vi "DB Execute.vi"(7 "table Name":string, 8 "error in (no error)":errorcluster, 11 "Db Reference":refnum<k24>) -> (0 "error out":errorcluster, 2 "Data":string[][](array[string]), 3 "Db Reference":refnum<k24>)   [LabVIEW 2020]
uses:
  D:/Labview/Auto Run Screen/Source Code/Database/Support/dbquery.dll
  Support/dbquery.dll
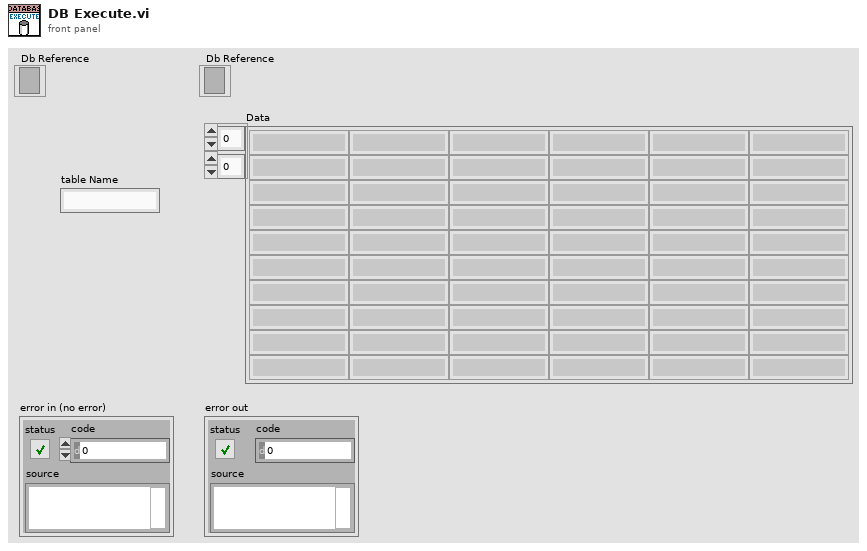
[diagram p1: front panel]
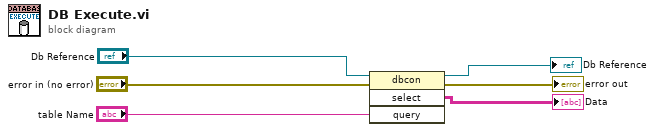
[diagram p0: block diagram]
diagram:
  n1 = invoke class="dbcon" method="select"(reference="Db Reference", error in="error in (no error)", "query"="table Name") -> (reference out=→"Db Reference":refnum<k24>, error out=→"error out":errorcluster, "select"=→"Data":string[][])  [unwired: 1 in, 1 out]
